vi "get channels.vi"(11 "user tag bus module configuration In":refnum<class "fixed channel tag bus module configuration.lvclass">) -> (2 "channels":refnum<class "TBM channel.lvclass">[](array[class]), 3 "user tag bus module configuration Out":refnum<class "fixed channel tag bus module configuration.lvclass">)   [LabVIEW 2013, in "fixed channel tag bus module configuration.lvclass"]
uses:
  fixed channel tag bus module configuration.lvclass
  <vilib>/NI/Tag Bus Module Framework/channel/TBM channel.lvclass
  fixed channel tag bus module configuration.lvclass/fixed channel tag bus module configuration.ctl
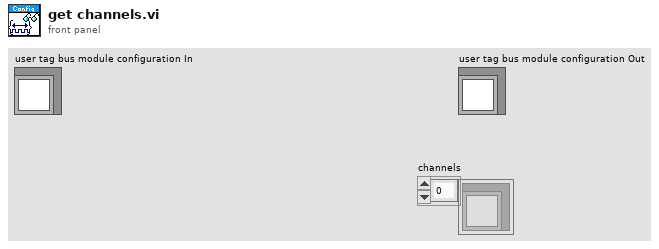
[diagram p1: front panel]
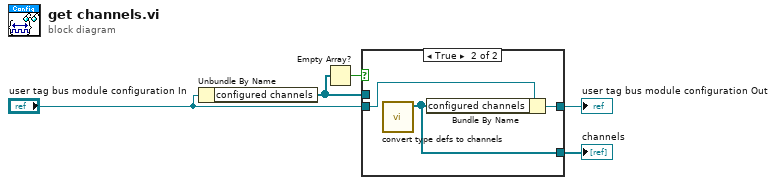
[diagram p0: block diagram]
diagram:
  n1 = Unbundle By Name("user tag bus module configuration In") -> ("configured channels"=w1:refnum<class "TBM channel.lvclass">[])
  n2 = Empty Array?(array=w1) -> (empty?=w2:bool)
  n3 = case shown="True" w2 {
    tunnel: "user tag bus module configuration In" -> [w7 w10]
    tunnel: [w7 w9] -> w4
    tunnel: w1 -> [w6 _]
    tunnel: [w6 w8] -> w3
    frame False {
    }
    frame True {
      n4 = call "convert type defs to channels.vi"() -> ("Array out"=w8:refnum<class "TBM channel.lvclass">[])  [unwired: 10 in, 1 out]
      n5 = Bundle By Name(cluster=w10, "configured channels"=w8) -> (w9:refnum<class "fixed channel tag bus module configuration.lvclass">)
    }
  }
  "user tag bus module configuration Out" <- w4
  "channels" <- w3
